vi "Configure Calibration.vi"(0 "VISA resource name":refnum<visa-resource-name>, 1 "Port 1 (1)":i32=1, 2 "Port 2 (1)":i32=1, 3 "Port 3 (1)":i32=1, 5 "error in (no error)":errorcluster, 6 "Channel (1)":i32=1, 7 "Error Correction State (F: Disable)":bool, 8 "Cal Kit (1)":i32=1, 9 "Velocity Factor (1.0)":dbl=1.0 format="%.2f", 10 "Calibration Type (4: Full 2-port)":u16(ring)=4 items=["Open", "Short", "Through", "1-port", "Full 2-port"], 11 "Calibration Property Display (F: Disable)":bool, 13 "z0 (50.0)":dbl=50.0 format="%.3f") -> (14 "VISA resource name out":refnum<visa-resource-name>, 19 "error out":errorcluster)   [LabVIEW 2012, in "Tektronix TTR500 Series.lvlib"]
doc: "This VI configures calibration parameters."
uses:
  <instrlib>/Tektronix TTR500 Series/Tektronix TTR500 Series.lvlib
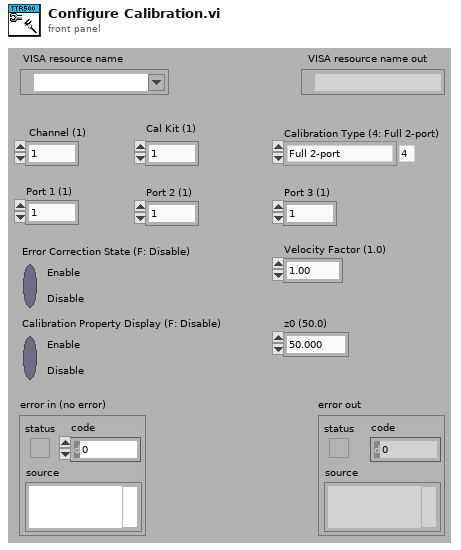
[diagram p1: front panel]
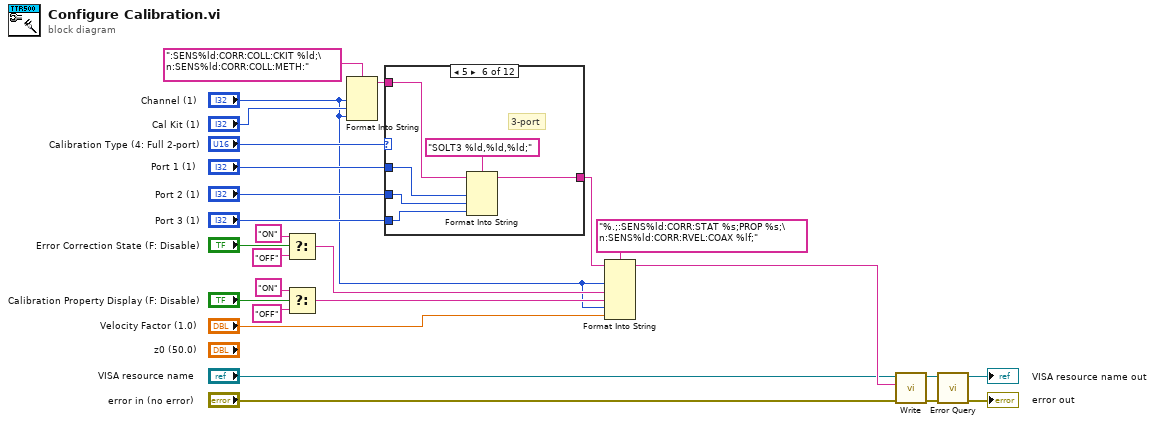
[diagram p0: block diagram]
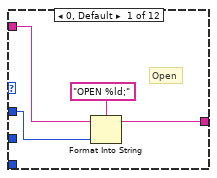
[diagram p2: hidden frame]
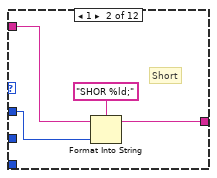
[diagram p3: hidden frame]
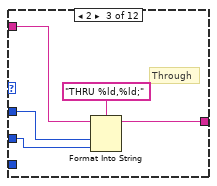
[diagram p4: hidden frame]
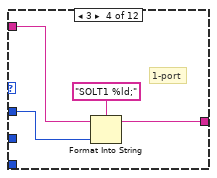
[diagram p5: hidden frame]
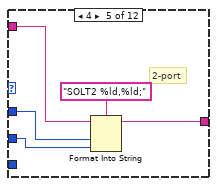
[diagram p6: hidden frame]
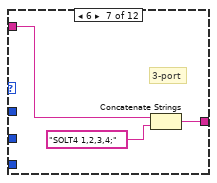
[diagram p7: hidden frame]
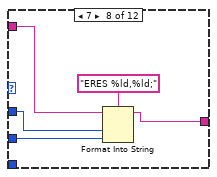
[diagram p8: hidden frame]
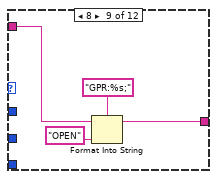
[diagram p9: hidden frame]
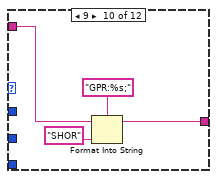
[diagram p10: hidden frame]
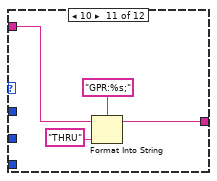
[diagram p11: hidden frame]
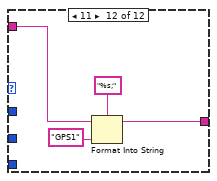
[diagram p12: hidden frame]
diagram:
  n1 = Select(t="ON", s="Error Correction State (F: Disable)", f="OFF") -> (s? t:f=w15:string)
  n2 = Select(t="ON", s="Calibration Property Display (F: Disable)", f="OFF") -> (s? t:f=w11:string)
  n3 = Format Into String(format string=":SENS%ld:CORR:COLL:CKIT %ld;\n:SENS%ld:CORR:COLL:METH:", "Channel (1)", "Cal Kit (1)", "Channel (1)") -> (resulting string=w22:string)  [unwired: 2 in, 1 out]
  n4 = case shown="5" "Calibration Type (4: Full 2-port)" {
    tunnel: "Port 1 (1)" -> [w29 w33 w38 w42 w47 w53 _ w60 _ _ _ _]
    tunnel: w22 -> [w28 w32 w37 w41 w46 w52 w57 w61 w64 w68 w72 w76]
    tunnel: [w27 w31 w36 w40 w45 w51 w55 w58 w63 w67 w71 w75] -> w4
    tunnel: "Port 2 (1)" -> [_ _ w35 _ w44 w50 _ w59 _ _ _ _]
    tunnel: "Port 3 (1)" -> [_ _ _ _ _ w49 _ _ _ _ _ _]
    frame 0, Default {
      # "Open"
      n5 = Format Into String(format string="OPEN %ld;", initial string=w28, w29) -> (resulting string=w27:string)  [unwired: 1 in, 1 out]
    }
    frame 1 {
      # "Short"
      n6 = Format Into String(format string="SHOR %ld;", initial string=w32, w33) -> (resulting string=w31:string)  [unwired: 1 in, 1 out]
    }
    frame 2 {
      # "Through"
      n7 = Format Into String(format string="THRU %ld,%ld;", initial string=w37, w38, w35) -> (resulting string=w36:string)  [unwired: 1 in, 1 out]
    }
    frame 3 {
      # "1-port"
      n8 = Format Into String(format string="SOLT1 %ld;", initial string=w41, w42) -> (resulting string=w40:string)  [unwired: 1 in, 1 out]
    }
    frame 4 {
      # "2-port"
      n9 = Format Into String(format string="SOLT2 %ld,%ld;", initial string=w46, w47, w44) -> (resulting string=w45:string)  [unwired: 1 in, 1 out]
    }
    frame 5 {
      # "3-port"
      n10 = Format Into String(format string="SOLT3 %ld,%ld,%ld;", initial string=w52, w53, w50, w49) -> (resulting string=w51:string)  [unwired: 1 in, 1 out]
    }
    frame 6 {
      # "3-port"
      n11 = Concatenate Strings(w57, "SOLT4 1,2,3,4;" ("format string")) -> (w55:string)
    }
    frame 7 {
      n12 = Format Into String(format string="ERES %ld,%ld;", initial string=w61, w60, w59) -> (resulting string=w58:string)  [unwired: 1 in, 1 out]
    }
    frame 8 {
      n13 = Format Into String(format string="GPR:%s;", initial string=w64, "OPEN" ("input 1")) -> (resulting string=w63:string)  [unwired: 1 in, 1 out]
    }
    frame 9 {
      n14 = Format Into String(format string="GPR:%s;", initial string=w68, "SHOR" ("input 1")) -> (resulting string=w67:string)  [unwired: 1 in, 1 out]
    }
    frame 10 {
      n15 = Format Into String(format string="GPR:%s;", initial string=w72, "THRU" ("input 1")) -> (resulting string=w71:string)  [unwired: 1 in, 1 out]
    }
    frame 11 {
      n16 = Format Into String(format string="%s;", initial string=w76, "GPS1" ("input 1")) -> (resulting string=w75:string)  [unwired: 1 in, 1 out]
    }
  }
  n17 = Format Into String(format string="%.;:SENS%ld:CORR:STAT %s;PROP %s;\n:SENS%ld:CORR:RVEL:COAX %lf;", initial string=w4, "Channel (1)", w15, w11, "Channel (1)", "Velocity Factor (1.0)") -> (resulting string=w3:string)  [unwired: 1 in, 1 out]
  n18 = call <instrlib>:"Write.vi"("error in (no error)"="error in (no error)", "String ()"=w3, "VISA resource name"="VISA resource name") -> ("error out"=w7:errorcluster, "VISA resource name out"=w8:refnum<visa-resource-name>)  [unwired: 6 in, 1 out]
  n19 = call <instrlib>:"Error Query.vi"("error in (no error)"=w7, "VISA resource name"=w8) -> ("error out"=→"error out":errorcluster, "VISA resource name out"=→"VISA resource name out":refnum<visa-resource-name>)  [unwired: 6 in, 2 out]
